vi "Add Tag.vi"(8 "error in (no error)":errorcluster, 10 "Tag":string, 11 "FeedItem.lvclass in":refnum<class "FeedItem.lvclass">) -> (0 "error out":errorcluster, 3 "FeedItem.lvclass out":refnum<class "FeedItem.lvclass">)   [LabVIEW 2020, in "FeedItem.lvclass"]
uses:
  <vilib>/NI_RSS/FeedItem/FeedItem.lvclass
  <vilib>/NI_RSS/FeedItem/FeedItem.lvclass/FeedItem.ctl
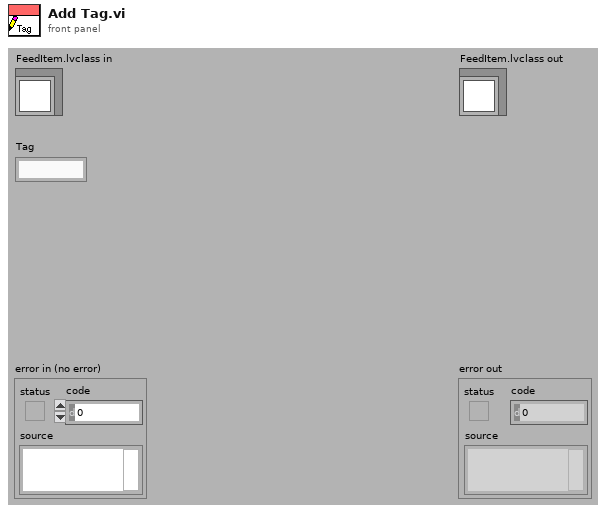
[diagram p1: front panel]
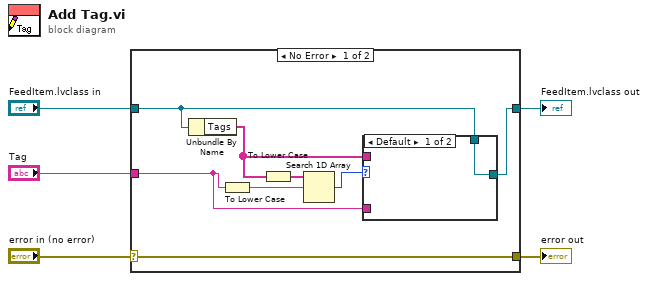
[diagram p0: block diagram]
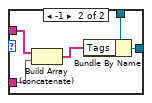
[diagram p2: hidden frame]
diagram:
  n1 = case shown="No Error" "error in (no error)" {
    selector: "error in (no error)" -> [w13 w20]
    tunnel: [w13 w20] -> w4
    tunnel: [w12 w21] -> w2
    tunnel: "FeedItem.lvclass in" -> [w11 w21]
    tunnel: "Tag" -> [w6 _]
    frame No Error {
      n2 = Unbundle By Name(w11) -> ("Tags"=w7:string[])
      n3 = To Lower Case(string=w6) -> (all lower case string=w9:string)
      n4 = To Lower Case(string=w7) -> (all lower case string=w10:string[])
      n5 = Search 1D Array(1D array=w10, element=w9) -> (index of element=w8:i32)  [unwired: 1 out]
      n6 = case shown="Default" w8 {
        tunnel: [w14 w19] -> w12
        tunnel: w11 -> [w14 w18]
        tunnel: w7 -> [_ w17]
        tunnel: w6 -> [_ w16]
        frame Default {
        }
        frame -1 {
          n7 = Build Array (concatenate)(w17, w16) -> (w15:string[])
          n8 = Bundle By Name(cluster=w18, "Tags"=w15) -> (w19:refnum<class "FeedItem.lvclass">)
        }
      }
    }
    frame Error {
    }
  }
  "error out" <- w4
  "FeedItem.lvclass out" <- w2
